vi "Search NaN_Inf (SubVI).vi"(1 "in":string[](array[string])) -> (0 "out":string[](array[string]))   [LabVIEW 2014]
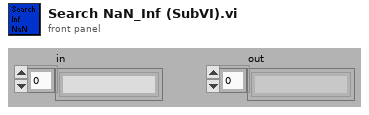
[diagram p1: front panel]
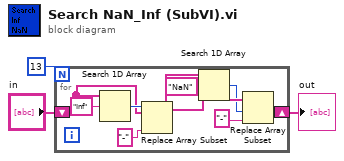
[diagram p0: block diagram]
diagram:
  n1 = for {
    N: 13 -> [_]
    shift-right: [w4] -> w2
    shift-left: "in" -> [w5]
    n2 = Search 1D Array(1D array=w5, element="Inf") -> (index of element=w10:i32)  [unwired: 1 in]
    n3 = Replace Array Subset(array=w5, new element="-" ("new element/subarray"), index=w10) -> (w7:string[])
    n4 = Search 1D Array(1D array=w7, element="NaN") -> (index of element=w6:i32)  [unwired: 1 in]
    n5 = Replace Array Subset(array=w7, new element="-" ("new element/subarray"), index=w6) -> (w4:string[])
  }
  "out" <- w2
